vi "Write Ignition Time.vi"(2 "error in (no error)":errorcluster, 3 "file path":path) -> (0 "error out":errorcluster, 1 "tdms file out":refnum<k34>)   [LabVIEW 2018]
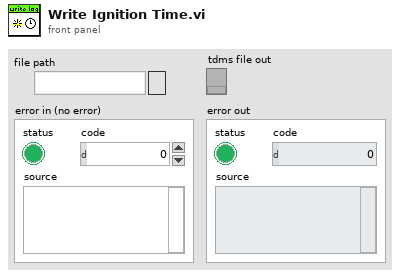
[diagram p1: front panel]
types:
  T1 = enum16{"open", "open or create", "create or replace", "create", "open (read-only)"}
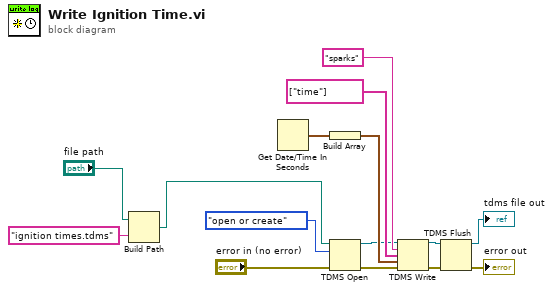
[diagram p0: block diagram]
diagram:
  n1 = Build Path(base path="file path", name or relative path="ignition times.tdms") -> (appended path=w2:path)
  n2 = Get Date/Time In Seconds() -> (seconds since 1Jan1904=w15:timestamp)
  n3 = Build Array(w15) -> (w14:timestamp[])
  n4 = TDMS Open(8:"error in (no error)", 10:T1."open or create" ("operation (0:open)"), 11:w2) -> (0:w5:errorcluster, 3:w6:refnum<k34>)  [unwired: 4 in]
  n5 = TDMS Write(0:w6, 5:"sparks" ("group name in (Untitled)"), 7:string[] ["time"] ("channel name(s) in (Untitled)"), 9:w14, 11:w5) -> (4:w9:refnum<k34>, 15:w8:errorcluster)  [unwired: 1 in, 2 out]
  n6 = TDMS Flush(4:w8, 7:w9) -> (0:→"error out":errorcluster, 3:→"tdms file out":refnum<k34>)
